vi "Configure Modules from Switches JSON.vi"() -> ()   [LabVIEW 2019]
uses:
  SubVIs/SLSC Switch Offline Configuration Information.ctl
  NationalInstruments.VeriStand.SystemDefinitionAPI
  <vilib>/addons/VeriStand Custom Device Scripting APIs/SLSC Switch/VeriStand SLSC Scripting API/VeriStand SLSC Scripting.lvlib
  <vilib>/addons/VeriStand Custom Device Scripting APIs/SLSC Switch/Scripting/SLSC Switch Scripting.lvlib
  SLSC Switch Examples.lvlib
panel:
  in  "SLSC Chassis Name or IP":string="slsc-12001-00000000"
  in  "Controller Name":string="Controller"
  in  "Custom Device Configuration":T1[](array[typedef])=[{"Switches JSON File"=path "C:/Program Files (x86)/National Instruments/Shared/NI-SLSC Switch/Modules/SLSC-12251-switches.json", "Slot Number"=2, "Model"="SLSC-12251"}]
  in  "Output System Definition file":path=path "System Definition Files/Scripted SLSC Switch.nivssdf"
  in  "Input System Definition File":path=path "System Definition Files/Base with SLSC Chassis.nivssdf"
  # "Overview: Demonstrates using the SLSC Switch custom device scripting API to configure instances of the custom device without requiring the hardware be present. By default, the configuration is for an NI SLSC-12251.\n\nInstructions:\n1. Browse to the system definition file to be used as input.\n2. Browse to a path to save the system definition file as output. This may be the same as the input file.\n3. Set the name of the controller in the system definition file that contains the SLSC Chassis\nand the SLSC Chassis identifier used in the system definition file. \n4. Select the slot number, model number, and resource/device name to script into the system definition file. \n5. Browse to the JSON file containing the switch definition, typically provided by the vendor.\n6. Repeat steps 4. and 5. for each custom device you wish to configure\n7. Run the VI and verify its results."
  # "System Definition Files"
  # "SLSC Chassis"
  # "Custom Device Configuration"
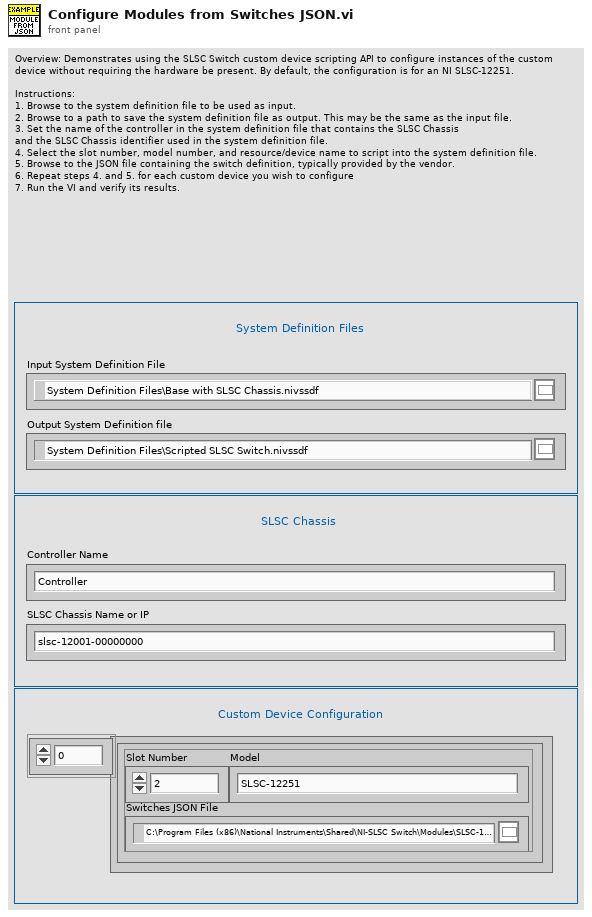
[diagram p1: front panel]
types:
  T1 = typedef "SLSC Switch Examples.lvlib/SLSC Switch Offline Configuration Information.ctl" = cluster{"Switches JSON File":path, "Slot Number":u32, "Model":string}
  T2 = typedef "Custom Device API.lvlib/Custom Device Item Ref.ctl" = u64
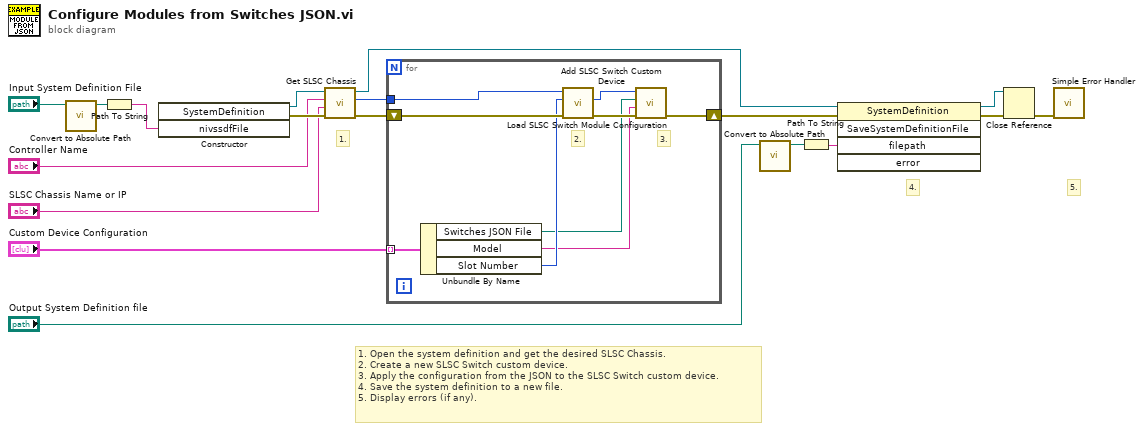
[diagram p0: block diagram]
diagram:
  # "1."
  # "4."
  # "5."
  # "1. Open the system definition and get the desired SLSC Chassis.\n2. Create a new SLSC Switch custom device.\n3. Apply the configuration from the JSON to the SLSC Switch custom device.\n4. Save the system definition to a new file.\n5. Display errors (if any)."
  n1 = call "Convert to Absolute Path.vi"("System Definition File"="Input System Definition File") -> ("Absolute Path"=w2:path)  [unwired: 10 in]
  n2 = Path To String(path=w2) -> (string=w11:string)
  n3 = constructor class="SystemDefinition"("nivssdfFile"=w11) -> (reference out=w9:refnum<k24>, error out=w10:errorcluster)  [unwired: 3 in, 2 out]
  n4 = call <vilib>:"Get SLSC Chassis.vi"("error in (no error)"=w10, "SLSC Chassis Name or IP"="SLSC Chassis Name or IP", "Target Name"="Controller Name", "SysDef in"=w9) -> ("error out"=w5:errorcluster, "SLSC Chassis"=w4:u64, "SysDef out"=w3:refnum<k24>)  [unwired: 4 in, 1 out]
  n5 = for {
    shift-right: [w23] -> w14
    shift-left: w5 -> [w25]
    tunnel: "Custom Device Configuration" -> [w27] mode=indexing
    tunnel: w4 -> [w26]
    # "3."
    # "2."
    n6 = Unbundle By Name(w27) -> ("Switches JSON File"=w20:path, "Model"=w19:string, "Slot Number"=w21:u32)
    n7 = call <vilib>:"Add SLSC Switch Custom Device.vi"("error in"=w25, "slot number"=w21, "slsc chassis in"=w26) -> ("error out"=w24:errorcluster, "slsc switch custom device"=w22:T2)  [unwired: 6 in, 1 out]
    n8 = call <vilib>:"Load SLSC Switch Module Configuration.vi"("error in"=w24, "product name"=w19, "switches json file"=w20, "slsc switch custom device in"=w22) -> ("error out"=w23:errorcluster)  [unwired: 6 in, 1 out]
  }
  n9 = call "Convert to Absolute Path.vi"("System Definition File"="Output System Definition file") -> ("Absolute Path"=w1:path)  [unwired: 10 in]
  n10 = Path To String(path=w1) -> (string=w18:string)
  n11 = invoke class="SystemDefinition" method="SaveSystemDefinitionFile"(reference=w3, error in=w14, "filepath"=w18) -> (reference out=w16:refnum<k24>, error out=w17:errorcluster)  [unwired: 2 in, 3 out]
  n12 = Close Reference(reference=w16, error in (no error)=w17) -> (error out=w13:errorcluster)
  n13 = call <vilib>:"Simple Error Handler.vi"("error in (no error)"=w13) -> ()  [unwired: 1 in, 8 out]
